vi "Assign seats.vi"(8 "error in":errorcluster, 10 "ref. Table":refnum<vi>, 11 "Table in":refnum<class "Table.lvclass">) -> (0 "error out":errorcluster, 3 "Table out":refnum<class "Table.lvclass">)   [LabVIEW 2023, in "Table.lvclass"]
uses:
  Table.lvclass
  C:/Program Files (x86)/National Instruments/LabVIEW 2023/vi.lib/addons/_Workers/Library/Classes/Worker/Worker.lvclass
  Table.lvclass/Table.ctl
  <vilib>/Utility/miscctls.llb/LVRectTypeDef.ctl
  <vilib>/addons/_Workers/Library/Classes/Callback Message/Enqueue and Collect.vi
  Philosopher/Philosopher.lvclass
  <vilib>/addons/_Workers/Library/Classes/Callback Message/Callback Message.lvclass
  C:/Program Files (x86)/National Instruments/LabVIEW 2023/vi.lib/addons/_Workers/Library/Classes/Workers Object/Workers Object.lvclass
  C:/Projects/DPP Workers/Workers/Table/Table.lvclass
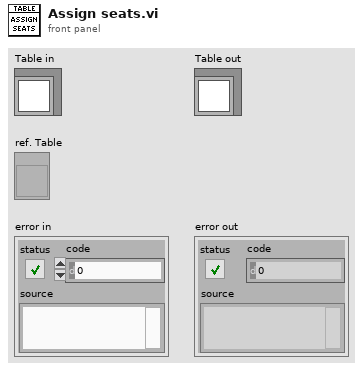
[diagram p1: front panel]
types:
  T1 = typedef "LVRectTypeDef.ctl" = cluster{"Left":i16, "Top":i16, "Right":i16, "Bottom":i16}
  T2 = typedef "Workers.lvlib/Case Label.ctl" = string
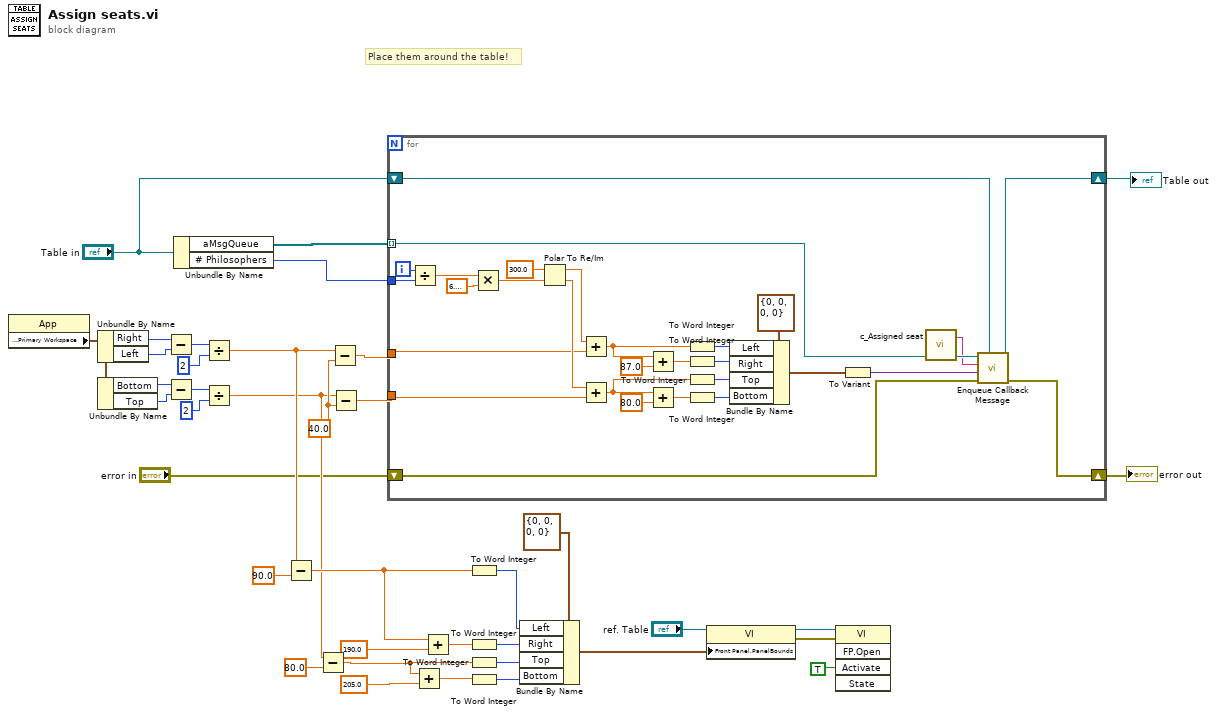
[diagram p0: block diagram]
diagram:
  w29 = 40.0 ("y")
  # "Place them around the table!"
  n1 = property on="Property Node" class="App"() -> ("Display:Primary Workspace"=w34:T1)  [unwired: 2 in, 2 out]
  n2 = Unbundle By Name(w34) -> ("Right"=w38:i16, "Left"=w37:i16)
  n3 = Unbundle By Name(w34) -> ("Bottom"=w31:i16, "Top"=w30:i16)
  n4 = Subtract(x=w38, y=w37) -> (x-y=w36:i16)
  n5 = Subtract(x=w31, y=w30) -> (x-y=w32:i16)
  n6 = Unbundle By Name("Table in") -> ("aMsgQueue"=w27:refnum<class "Message Queue.lvclass">[], "# Philosophers"=w28:i32)
  n7 = Divide(x=w36, y=i16 2) -> (x/y=w9:dbl)
  n8 = Divide(x=w32, y=i16 2) -> (x/y=w4:dbl)
  n9 = Subtract(x=w9, y=90.0) -> (x-y=w7:dbl)
  n10 = Subtract(x=w4, y=80.0) -> (x-y=w3:dbl)
  n11 = Subtract(x=w9, y=w29) -> (x-y=w6:dbl)
  n12 = Subtract(x=w4, y=w29) -> (x-y=w11:dbl)
  n13 = for {
    tunnel: w27 -> [w46] mode=indexing
    tunnel: w28 -> [w55]
    tunnel: w11 -> [w54]
    tunnel: w6 -> [w53]
    shift-right: [w41] -> w25
    shift-left: "Table in" -> [w42]
    shift-right: [w39] -> w1
    shift-left: "error in" -> [w40]
    i -> [w56]
    n14 = Divide(x=w56, y=w55) -> (x/y=w67:dbl)
    n15 = Multiply(x=w67, y=6.283185307179586 ("Pi Multiplied By 2")) -> (x*y=w65:dbl)
    n16 = Polar To Re/Im(2:w65, 3:300.0 ("r")) -> (0:w62:dbl, 1:w63:dbl)
    n17 = Add(x=w63, y=w53) -> (x+y=w60:dbl)
    n18 = Add(x=w62, y=w54) -> (x+y=w52:dbl)
    n19 = Add(x=w60, y=87.0) -> (x+y=w51:dbl)
    n20 = Add(x=w52, y=80.0) -> (x+y=w58:dbl)
    n21 = To Word Integer(number=w60) -> (16bit integer=w50:i16)
    n22 = To Word Integer(number=w51) -> (16bit integer=w49:i16)
    n23 = To Word Integer(number=w52) -> (16bit integer=w48:i16)
    n24 = To Word Integer(number=w58) -> (16bit integer=w47:i16)
    n25 = Bundle By Name(cluster=T1 {"Left"=0, "Top"=0, "Right"=0, "Bottom"=0} ("Front Panel Window:Window Bounds"), "Left"=w50, "Right"=w49, "Top"=w48, "Bottom"=w47) -> (w45:T1)
    n26 = To Variant(anything=w45) -> (Variant=w44:variant)
    n27 = call "c_Assigned seat.vi"() -> ("Case Label"=w43:T2)  [unwired: 1 in]
    n28 = call-poly <vilib>:"Enqueue Callback Message.vi"("Worker"=w42, "error in"=w40, "Data"=w44, "Case Label"=w43, "Message Queue"=w46) -> ("error out"=w39:errorcluster, "dup Worker out"=w41:refnum<class "Table.lvclass">)  [unwired: 3 in, 2 out]
  }
  "Table out" <- w25
  "error out" <- w1
  n29 = Add(x=w3, y=205.0 ("Right")) -> (x+y=w13:dbl)
  n30 = Add(x=w7, y=190.0 ("Right")) -> (x+y=w17:dbl)
  n31 = To Word Integer(number=w7) -> (16bit integer=w19:i16)
  n32 = To Word Integer(number=w17) -> (16bit integer=w16:i16)
  n33 = To Word Integer(number=w3) -> (16bit integer=w18:i16)
  n34 = To Word Integer(number=w13) -> (16bit integer=w12:i16)
  n35 = Bundle By Name(cluster=T1 {"Left"=0, "Top"=0, "Right"=0, "Bottom"=0} ("Front Panel Window:Window Bounds"), "Left"=w19, "Right"=w16, "Top"=w18, "Bottom"=w12) -> (w21:T1)
  n36 = property on="Property Node" class="VI"(reference="ref. Table", "Front Panel.PanelBounds"=w21) -> (reference out=w10:refnum<vi>, error out=w23:errorcluster)  [unwired: 1 in]
  n37 = invoke on="Invoke Node" class="VI" method="FP.Open"(reference=w10, error in=w23, "Activate"=TRUE ("Activate?")) -> ()  [unwired: 2 in, 5 out]
